vi "Flatten.vi"(8 "error in":errorcluster, 9 "Command Data":T1 {"Time Stamp" format="%<%x %.3X>T"}) -> (0 "error out":errorcluster, 2 "Buffer":u8[](array[numeric]) format="%.0x")   [LabVIEW 2023, in "ConstellationCommand.lvlib"]
uses:
  ConstellationCommand.lvlib
  <vilib>/IlluminatedG/IG Protoc/LV-Proto/LV-Proto.lvlib
  Data.ctl
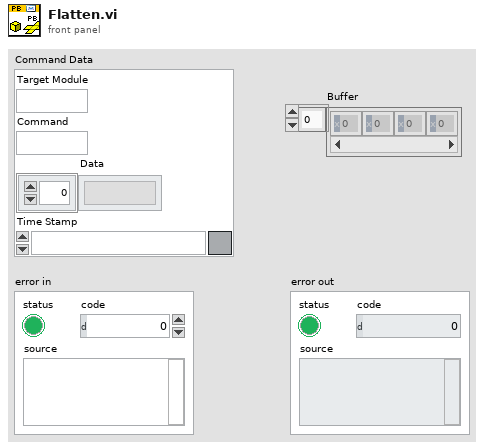
[diagram p1: front panel]
types:
  T1 = typedef "ConstellationCommand.lvlib/Data.ctl" = cluster{"Target Module":string, "Command":string, "Data":string[], "Time Stamp":timestamp}
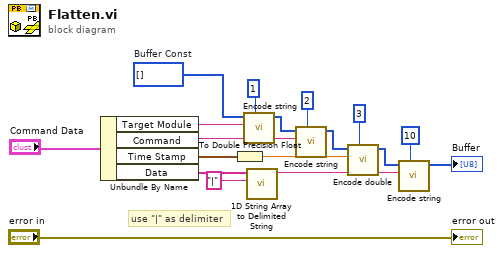
[diagram p0: block diagram]
diagram:
  w17 = u8[] []  # Buffer Const
  # "use \"|\" as delimiter"
  n1 = Unbundle By Name("Command Data") -> ("Target Module"=w16:string, "Command"=w14:string, "Time Stamp"=w8:timestamp, "Data"=w4:string[])
  n2 = To Double Precision Float(number=w8) -> (double precision float=w7:dbl)
  n3 = call <vilib>:"Encode string.vi"("Field Number"=1, "string"=w16, "Buffer in"=w17) -> ("Buffer"=w12:u8[])  [unwired: 8 in]
  n4 = call <vilib>:"1D String Array to Delimited String.vi"("delimiter"="|", "string array"=w4) -> ("delimited string"=w2:string)  [unwired: 9 in]
  n5 = call <vilib>:"Encode string.vi"("Field Number"=2, "string"=w14, "Buffer in"=w12) -> ("Buffer"=w10:u8[])  [unwired: 8 in]
  n6 = call <vilib>:"Encode double.vi"("Field Number"=3, "double"=w7, "Buffer in"=w10) -> ("Buffer"=w6:u8[])  [unwired: 8 in]
  n7 = call <vilib>:"Encode string.vi"("Field Number"=10, "string"=w2, "Buffer in"=w6) -> ("Buffer"=→"Buffer":u8[])  [unwired: 8 in]
  "error out" <- "error in"
